vi "MeasureRMS.vi"(9 "input cluster":T1) -> (2 "AC estimate (Vrms)":dbl format="%0.2f")   [LabVIEW 2014]
uses:
  <vilib>/Analysis/NI_AALPro.lvlib
panel:
  out "data":dynamicdata(graph)
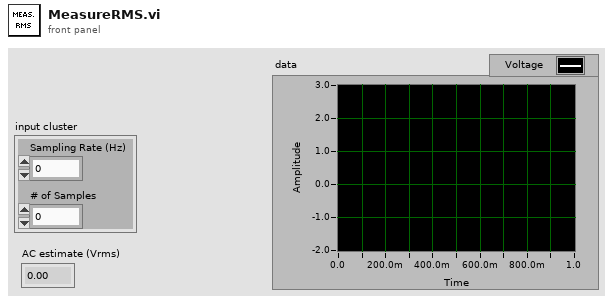
[diagram p1: front panel]
types:
  T1 = cluster{"Sampling Rate (Hz)":dbl, "# of Samples":dbl}
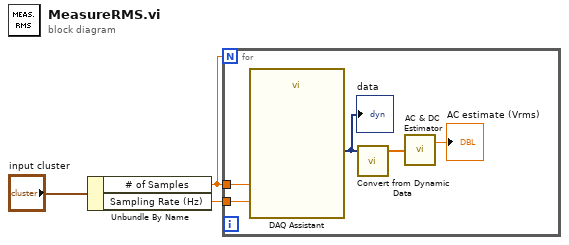
[diagram p0: block diagram]
diagram:
  n1 = Unbundle By Name("input cluster") -> ("# of Samples"=w2:dbl, "Sampling Rate (Hz)"=w1:dbl)
  n2 = for {
    N: w2 -> [_]
    tunnel: w2 -> [w7]
    tunnel: w1 -> [w6]
    n3 = call "DAQ Assistant"("rate"=w6, "number of samples"=w7) -> ("data"=w4:dynamicdata)  [unwired: 15 in, 2 out]
    "data" <- w4
    n4 = call "Convert from Dynamic Data"("Dynamic Data Type"=w4) -> ("Array"=w8:dbl[])  [unwired: 3 in]
    n5 = call <vilib>:"AC & DC Estimator.vi"("Signal (V)"=w8) -> ("AC estimate (Vrms)"=→"AC estimate (Vrms)":dbl)  [unwired: 1 out]
  }
